vi "DoE_Control_Main.vi"() -> ()   [LabVIEW 2015]
uses:
  --Controls and TypeDefs--/DoE_Control_Cluster.ctl
  <instrlib>/JULABO DeviceDriver/Examples/Julabo Serial Control.ctl
  <instrlib>/JULABO DeviceDriver/JULABO DeviceDriver.lvlib
  <vilib>/ptbypt/NI_PtbyPt.lvlib
panel:
  out "Producer Iteration":i32
  out "Error?":bool
  out "Error?":errorcluster
  out "error out":errorcluster
  out "Measurement Iteration":i32
  out "Consumer Iteration":i32
  out "Slave Data Cluster":T1={"Current DoE"=[], "SSI 1 Flow Rate"=0.0, "SSI 2 Flow Rate"=0.0, "FLOM 1 Flow Rate"=0.0, "FLOM 2 Flow Rate"=0.0, "Pumps Running?"=FALSE, "Boolean 2"=FALSE, "Boolean 3"=FALSE, "Boolean 4"=FALSE, "At Equilibrium?"=FALSE, "Script Running?"=FALSE, "Current Script Iteration"=0.0, "Total Script Iterations"=0.0, "FLOM Pumps VISA"="COM2", "SSI 1 Pump VISA"="COM76", "SSI 2 Pump VISA"="COM74", "Huber Unistat VISA"="COM1", "SSI 3 Pump VISA"="COM76", "SSI 4 Pump VISA"="COM76", "SSI 4 Flow Rate"=0.0, "SSI 3 Flow Rate"=0.0, "Flow Meter 1 Rate "=0.0, "Flow Meter 2 Rate"=0.0, "Flow Meter 3 Rate"=0.0, "Flow Meter 4 Rate"=0.0, "SSI 1 Flow Setpoint"=0.0, "SSI 2 Flow Setpoint"=0.0, "SSI 3 Flow Setpoint"=0.0, "SSI 4 Flow Setpoint"=0.0, "Temperature Setpoint"=0.0, "Flow meter 3 COM"=17, "Flow meter 5 COM"=18, "Flow meter 4 COM"=19, "Flow meter 2 COM"=16, "Flow meter 1 COM"=15, "Unit"=enum."PSI", "Pressure COM"="COM6", "Julabo Setpoint"=0.0, "Julabo Control"=enum."Internal", "Overtemp"=50.0, "Subtemp"=-20.0, "HeatMax"=50, "CoolMax"=-100, "InternMax"=50.0, "InternMin"=0.0, "Upper Bandlimit"=100.0, "Lower Bandlimit"=0.0, "Julabo CF41 VISA"="COM3", "Xp (0.6K) Int"=0.6, "Tn (3s) Int"=3, "Tv (0s) Int"=0, "Dynamic (0: aperiodic) Int"=enum."aperiodic", "Xp (0.6K) Ext"=0.6, "Tn (3s) Ext"=3, "Tv (0s) Ext"=0, "XpU (0.6K) Ext"=0.6, "Julabo Serial Configuration"={"Baud Rate"=4800, "Parity"=2, "Data Bits"=7, "Stop Bits"=10, "Flow Control"=2}} {"Julabo Serial Configuration"."Flow Control" items=["None", "XON/XOFF", "RTS/CTS", "XON/XOFF & RTS/CTS", "DTR/DSR", "XON/XOFF & DTR/DSR"]; "Julabo Serial Configuration"."Stop Bits" items=["1.0"=10, "1.5"=15, "2.0"=20]; "Julabo Serial Configuration"."Data Bits" items=["7"=7, "8"=8]; "Julabo Serial Configuration"."Parity" items=["None", "Odd", "Even", "Mark", "Space"]; "Julabo Serial Configuration"."Baud Rate" items=["300"=300, "600"=600, "1200"=1200, "2400"=2400, "4800"=4800, "9600"=9600, "19200"=19200]; "XpU (0.6K) Ext" min=0.1 max=99.9; "Tv (0s) Ext" max=999; "Tn (3s) Ext" min=3 max=9999; "Xp (0.6K) Ext" min=0.1 max=99.9; "Tv (0s) Int" max=999; "Tn (3s) Int" min=3 max=9999; "Xp (0.6K) Int" min=0.1 max=99.9; "Lower Bandlimit" min=0.0 max=200.0; "Upper Bandlimit" min=0.0 max=200.0; "InternMin" format="%.2f"; "InternMax" format="%.2f"; "CoolMax" min=-100 max=0; "HeatMax" max=100; "Subtemp" format="%.2f"; "Overtemp" format="%.2f"; "Julabo Setpoint" format="%.2f"; "Current DoE" format="%0.3f"}
  in  "Sensor Readouts":T3(tab)
  out "Thermocouple T-Plots":T4(graph)
  in  "Apply Moving Average?":bool=TRUE
  out "dT/dt":cluster{"dx/dt":dbl, "dx/dt":dbl, "dx/dt":dbl}(graph)
  out "Flow Rate":T5(graph)
  out "dF/dt":T5(graph)
  in  "Apply dF/dt?":bool=TRUE
  out "Temp":T6(graph)
  out "Pressure":T7(graph)
  out "Internal Temp":dbl format="%.2f"
  out "Power":i8(slide) scale=-100.0..100.0
  out "Diagram":T8(graph)
  out "External Temp":dbl format="%.2f"
  out "Safety Temp":dbl
  out "Excess Temp Protection":dbl
  in  "Write to File?":bool
  in  "?":T9(tab)
  in  "Collect Spectra":bool
  out "Raman Spectrum":cluster{i32[], i32[]}[](graph)
  in  "Reset?":bool
  in  "Cancel Script":bool
  in  "Main Data Cluster":T1={"Current DoE"=[], "SSI 1 Flow Rate"=0.0, "SSI 2 Flow Rate"=0.0, "FLOM 1 Flow Rate"=0.0, "FLOM 2 Flow Rate"=0.0, "Pumps Running?"=FALSE, "Boolean 2"=FALSE, "Boolean 3"=FALSE, "Boolean 4"=FALSE, "At Equilibrium?"=FALSE, "Script Running?"=FALSE, "Current Script Iteration"=0.0, "Total Script Iterations"=0.0, "FLOM Pumps VISA"="COM2", "SSI 1 Pump VISA"="COM76", "SSI 2 Pump VISA"="COM74", "Huber Unistat VISA"="COM1", "SSI 3 Pump VISA"="COM76", "SSI 4 Pump VISA"="COM76", "SSI 4 Flow Rate"=0.0, "SSI 3 Flow Rate"=0.0, "Flow Meter 1 Rate "=0.0, "Flow Meter 2 Rate"=0.0, "Flow Meter 3 Rate"=0.0, "Flow Meter 4 Rate"=0.0, "SSI 1 Flow Setpoint"=0.0, "SSI 2 Flow Setpoint"=0.0, "SSI 3 Flow Setpoint"=0.0, "SSI 4 Flow Setpoint"=0.0, "Temperature Setpoint"=0.0, "Flow meter 3 COM"=17, "Flow meter 5 COM"=18, "Flow meter 4 COM"=19, "Flow meter 2 COM"=16, "Flow meter 1 COM"=15, "Unit"=enum."PSI", "Pressure COM"="COM6", "Julabo Setpoint"=0.0, "Julabo Control"=enum."Internal", "Overtemp"=50.0, "Subtemp"=-20.0, "HeatMax"=50, "CoolMax"=-100, "InternMax"=50.0, "InternMin"=0.0, "Upper Bandlimit"=100.0, "Lower Bandlimit"=0.0, "Julabo CF41 VISA"="COM3", "Xp (0.6K) Int"=0.6, "Tn (3s) Int"=3, "Tv (0s) Int"=0, "Dynamic (0: aperiodic) Int"=enum."aperiodic", "Xp (0.6K) Ext"=0.6, "Tn (3s) Ext"=3, "Tv (0s) Ext"=0, "XpU (0.6K) Ext"=0.6, "Julabo Serial Configuration"={"Baud Rate"=4800, "Parity"=2, "Data Bits"=7, "Stop Bits"=10, "Flow Control"=2}} {"Julabo Serial Configuration"."Flow Control" items=["None", "XON/XOFF", "RTS/CTS", "XON/XOFF & RTS/CTS", "DTR/DSR", "XON/XOFF & DTR/DSR"]; "Julabo Serial Configuration"."Stop Bits" items=["1.0"=10, "1.5"=15, "2.0"=20]; "Julabo Serial Configuration"."Data Bits" items=["7"=7, "8"=8]; "Julabo Serial Configuration"."Parity" items=["None", "Odd", "Even", "Mark", "Space"]; "Julabo Serial Configuration"."Baud Rate" items=["300"=300, "600"=600, "1200"=1200, "2400"=2400, "4800"=4800, "9600"=9600, "19200"=19200]; "XpU (0.6K) Ext" min=0.1 max=99.9; "Tv (0s) Ext" max=999; "Tn (3s) Ext" min=3 max=9999; "Xp (0.6K) Ext" min=0.1 max=99.9; "Tv (0s) Int" max=999; "Tn (3s) Int" min=3 max=9999; "Xp (0.6K) Int" min=0.1 max=99.9; "Lower Bandlimit" min=0.0 max=200.0; "Upper Bandlimit" min=0.0 max=200.0; "InternMin" format="%.2f"; "InternMax" format="%.2f"; "CoolMax" min=-100 max=0; "HeatMax" max=100; "Subtemp" format="%.2f"; "Overtemp" format="%.2f"; "Julabo Setpoint" format="%.2f"; "Current DoE" format="%0.3f"}
  in  "?":T10(tab)
  in  "Huber Unistat VISA":refnum<visa-resource-name>="COM1"
  in  "SSI 4 Pump VISA":refnum<visa-resource-name>="COM10"
  in  "SSI 2 Pump VISA 2":refnum<visa-resource-name>="COM8"
  in  "SSI 1 Pump VISA":refnum<visa-resource-name>="COM7"
  in  "FLOM Pumps VISA":refnum<visa-resource-name>="LPT1"
  in  "SSI 3 Pump VISA":refnum<visa-resource-name>="COM9"
  in  "Set COMs":bool
  out "Data_noRaman path":path caption="selected path"
  out "Data_Reactant 1 path":path caption="selected path"
  out "Data_Product path":path caption="selected path"
  out "Data_Reactant 3 path":path caption="selected path"
  out "Data_Reactant 2 path":path caption="selected path"
  out "Raman Data Path":T11
  in  "Flow meter 5 COM":u16=18
  in  "Flow meter 4 COM":u16=19
  in  "Flow meter 3 COM":u16=17
  in  "Flow meter 2 COM":u16=16
  in  "Flow meter 1 COM":u16=15
  in  "Unit":T12(ring)
  in  "Pressure COM":refnum<visa-resource-name>="COM6"
  in  "Julabo Serial Configuration":T2={"Baud Rate"=4800, "Parity"=2, "Data Bits"=7, "Stop Bits"=10, "Flow Control"=2} {"Flow Control" items=["None", "XON/XOFF", "RTS/CTS", "XON/XOFF & RTS/CTS", "DTR/DSR", "XON/XOFF & DTR/DSR"]; "Stop Bits" items=["1.0"=10, "1.5"=15, "2.0"=20]; "Data Bits" items=["7"=7, "8"=8]; "Parity" items=["None", "Odd", "Even", "Mark", "Space"]; "Baud Rate" items=["300"=300, "600"=600, "1200"=1200, "2400"=2400, "4800"=4800, "9600"=9600, "19200"=19200]}
  in  "Julabo CF41 VISA":refnum<visa-resource-name>="COM11"
  in  "RS485-Address (128: RS232)":u32=128
  in  "Create DoE":bool
  out "file write cancelled":bool caption="cancelled"
  out "written file already exists (and overwritten)":bool caption="exists"
  in  "Input DoE Values":string[][](table)
  in  "Load DoE":bool
  out "Current DoE":dbl[][](array[numeric]) format="%0.3f"
  out "DoE Filename":path
  in  "Get Current DoE":bool
  in  "Stop-Start SSI 4":bool
  in  "Stop-Start SSI 3":bool
  in  "Edit or Run/Stop SSI 4":string(combo)="Run/Stop"
  in  "Edit or Run/Stop SSI 3":string(combo)="Run/Stop"
  in  "Pump 4 (Green)?":bool
  in  "Pump 3 (Yellow)?":bool
  in  "SSI  4 (Green)":dbl
  in  "SSI  3 (Yellow)":dbl
  in  "SSI  1 (Red)":dbl
  in  "Manual Pump Control?":bool
  in  "SSI  2 (Blue)":dbl
  in  "Pump 1 (Red)?":bool
  in  "Pump 2 (Blue)?":bool
  in  "Edit or Run/Stop SSI 2":string(combo)="Run/Stop"
  in  "Edit or Run/Stop SSI 1":string(combo)="Run/Stop"
  in  "Stop-Start SSI 1":bool
  in  "Stop-Start SSI 2":bool
  in  "FLOM 1":dbl min=0.0 max=9900.0 step=1.0
  in  "FLOM 2":dbl min=0.0 max=9900.0 step=1.0
  in  "FLOM 1?":bool
  in  "FLOM 2?":bool
  in  "Stop   Start FLOM 1":bool
  in  "Stop   Start FLOM 2":bool
  in  "Edit Values, or Run Flow? FLOM 2":string(combo)="Run/Stop"
  in  "Edit Values, or Run Flow? FLOM 1":string(combo)="Run/Stop"
  out "SSI  2  (Blue) Feedback":i32 format="%.2f"
  out "SSI  1  (Red) Feedback":i32 format="%.2f"
  out "SSI  3  (Yellow) Feedback":i32 format="%.2f"
  out "SSI  4  (Green) Feedback":i32 format="%.2f"
  in  "Manual Temp Control?":bool
  in  "Julabo Setpoint":dbl format="%.2f"
  in  "Julabo Control Type":enum16{"Internal", "External"}(ring)
  in  "JulaboStartStop":bool
  in  "btnAdjustWarningLevels":bool
  in  "btnAdjustCapacityLevels":bool
  in  "btnAdjustBandLimits":bool
  in  "btnAdjustInternalTempLimits":bool
  in  "btnAdjustInternalControlParams":bool
  in  "btnAdjustExternalControlParams":bool
  in  "Xp (0.6K)":dbl=0.6 min=0.1 max=99.9
  in  "Tn (3s)":u16=3 min=3 max=9999
  in  "Tv (0s)":u16 max=999
  in  "Dynamic (0: aperiodic)":enum16{"aperiodic", "standard"}(ring)
  in  "XpU (0.6K) Ext":dbl=0.6 min=0.1 max=99.9
  in  "Xp (0.6K) Ext":dbl=0.6 min=0.1 max=99.9
  in  "Tn (3s) Ext":u16=3 min=3 max=9999
  in  "Tv (0s) Ext":u16 max=999
  in  "Overtemp":dbl=50.0 format="%.2f"
  in  "Subtemp":dbl=-20.0 format="%.2f"
  in  "HeatMax":u8=50 max=100
  in  "CoolMax":i8=-100 min=-100 max=0
  in  "InternMax":dbl=50.0 format="%.2f"
  in  "InternMin":dbl format="%.2f"
  in  "Lower Bandlim":dbl min=0.0 max=200.0
  in  "Upper Bandlim":dbl=100.0 min=0.0 max=200.0
  in  "Run Current DoE":bool
  out "Current Experiment":dbl[](array[numeric])
  in  "Debugging / Send Command":string
  in  "Debug":bool
  out "Total Script Iterations":i32
  out "Total Script Iterations 2":dbl
  out "Current Script Iteration":dbl
  out "Program State":string
  in  "STOP":bool
  # "Most recent update: 4/13/2016 - JMW"
  # "Features To-Implement:\n\n- Yield Plotting and Analytics\n- Feedback Control based on Yield\n- Error Generation System\n     - for system and user safety"
  # "Notes:\n- when starting a DoE, either have both pumps and chiller on or off\n- Always use Stop Program rather than the LabView stop button, else the Sensirion DLL\n   calls will error out and LabView must be restarted"
  # "Julabo"
  # "Limits"
  # "PID Control Parameters"
  # "Julabo"
  # "Limits"
  # "PID Control Parameters"
  # "control type \n(hold, equil)"
  # "SSI 1"
  # "SSI 2"
  # "SSI 3"
  # "SSI 4"
  # "Temp"
  # "Time"
  # "FLOM 1"
  # "FLOM 2"
  # "hold - time\nequil - watch var, deriv.\nequil timeout\n\nadd setpoint limit control"
  # "SSI 1"
  # "SSI 2"
  # "SSI 3"
  # "SSI 4"
  # "FLOM 1"
  # "FLOM 2"
  # "Temp"
  # "Time"
  # "All flow rates in increments of 10uL/min"
  # "Note: don't repeatedly turn off and on temperature control as this can wear out the compressor too rapidly according to Unistat\nManual"
  # "Gratuitously Large Power Button"
  # "Internal parameters"
  # "External parameters"
  # "Time"
  # "Control"
  # "Temp"
  # "SSI 1"
  # "SSI 2"
  # "SSI 3"
  # "SSI 4"
  # "FLOM 1"
  # "FLOM 2"
  # "uL/min , degrees C, seconds"
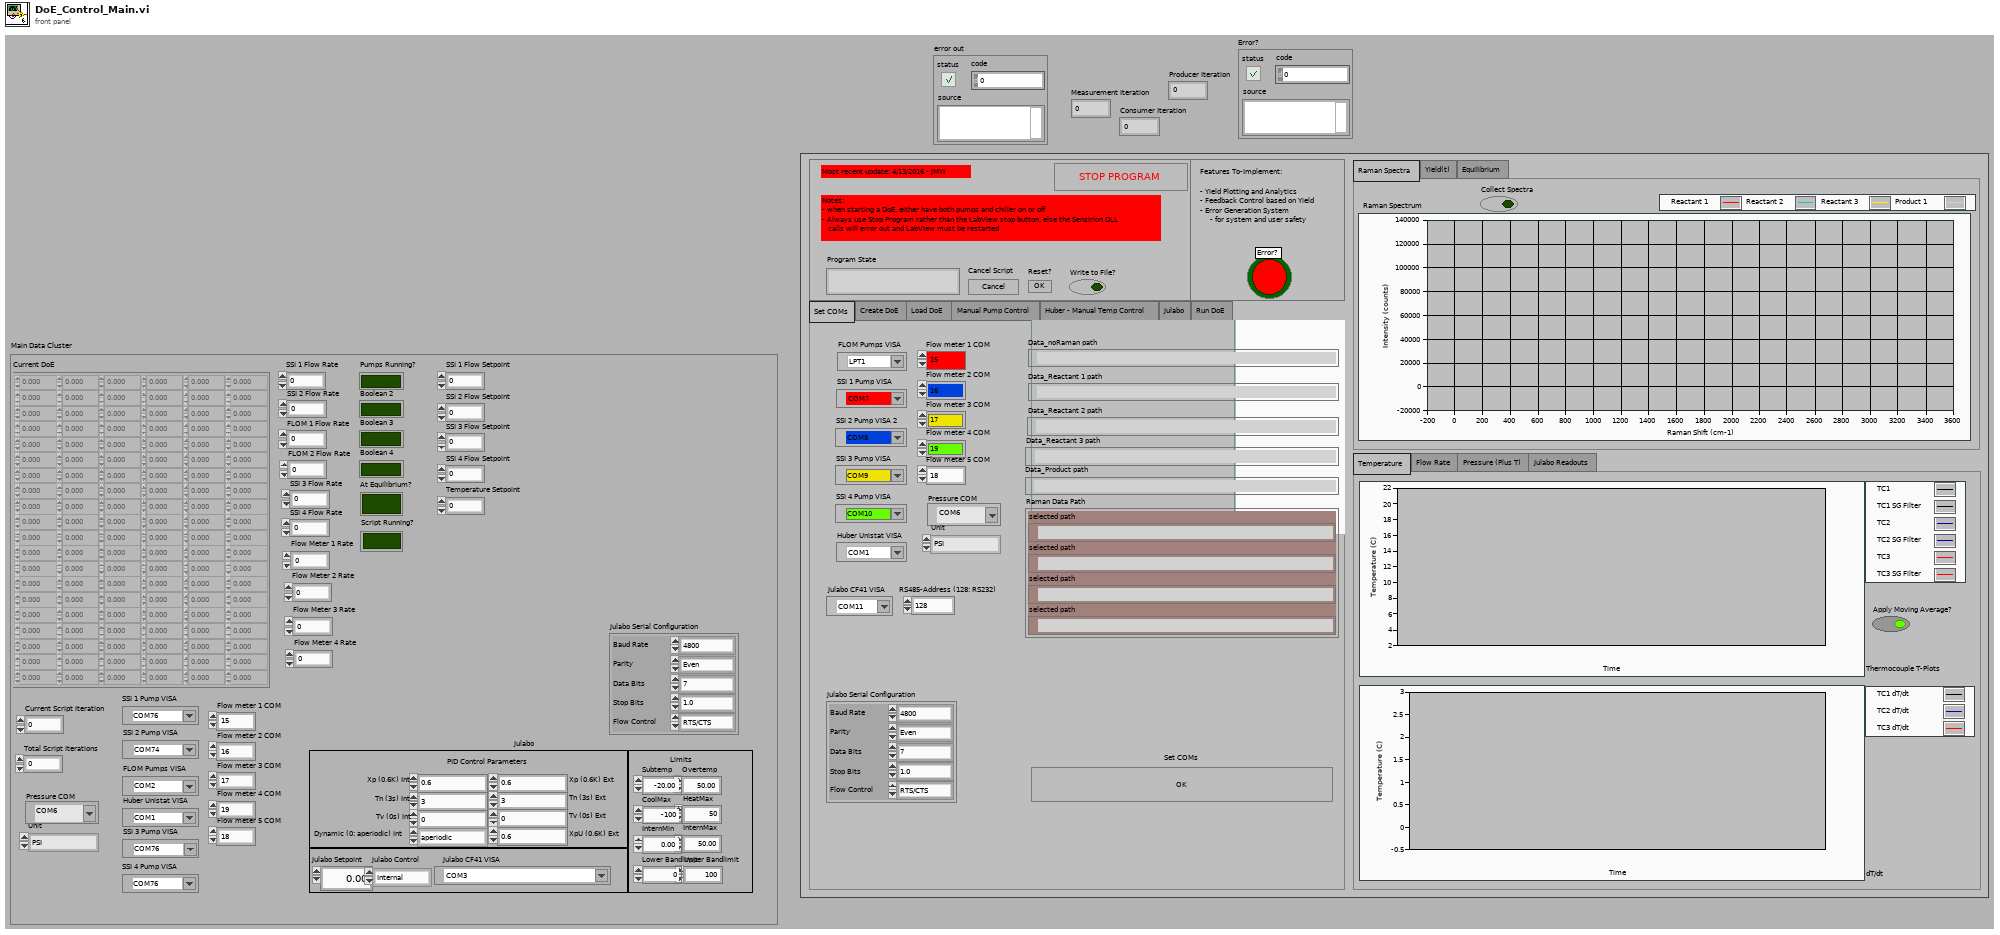
[diagram p1: front panel]
types:
  T1 = typedef "DoE_Control_Cluster.ctl" = cluster{"Current DoE":dbl[][], "SSI 1 Flow Rate":dbl, "SSI 2 Flow Rate":dbl, "FLOM 1 Flow Rate":dbl, "FLOM 2 Flow Rate":dbl, "Pumps Running?":bool, "Boolean 2":bool, "Boolean 3":bool, "Boolean 4":bool, "At Equilibrium?":bool, "Script Running?":bool, "Current Script Iteration":dbl, "Total Script Iterations":dbl, "FLOM Pumps VISA":refnum<visa-resource-name>, "SSI 1 Pump VISA":refnum<visa-resource-name>, "SSI 2 Pump VISA":refnum<visa-resource-name>, "Huber Unistat VISA":refnum<visa-resource-name>, "SSI 3 Pump VISA":refnum<visa-resource-name>, "SSI 4 Pump VISA":refnum<visa-resource-name>, "SSI 4 Flow Rate":dbl, "SSI 3 Flow Rate":dbl, "Flow Meter 1 Rate ":dbl, "Flow Meter 2 Rate":dbl, "Flow Meter 3 Rate":dbl, "Flow Meter 4 Rate":dbl, "SSI 1 Flow Setpoint":dbl, "SSI 2 Flow Setpoint":dbl, "SSI 3 Flow Setpoint":dbl, "SSI 4 Flow Setpoint":dbl, "Temperature Setpoint":dbl, "Flow meter 3 COM":u16, "Flow meter 5 COM":u16, "Flow meter 4 COM":u16, "Flow meter 2 COM":u16, "Flow meter 1 COM":u16, "Unit":enum16{"PSI", "Bar", "cm H2O", "ft H2O", "hectoPascal", "in Hg", "in H2O", "kiloPascal", "milliBar", "mmHg", "MegaPascal", "Numeric Pressure"}, "Pressure COM":refnum<visa-resource-name>, "Julabo Setpoint":dbl, "Julabo Control":enum16{"Internal", "External"}, "Overtemp":dbl, "Subtemp":dbl, "HeatMax":u8, "CoolMax":i8, "InternMax":dbl, "InternMin":dbl, "Upper Bandlimit":dbl, "Lower Bandlimit":dbl, "Julabo CF41 VISA":refnum<visa-resource-name>, "Xp (0.6K) Int":dbl, "Tn (3s) Int":u16, "Tv (0s) Int":u16, "Dynamic (0: aperiodic) Int":enum16{"aperiodic", "standard"}, "Xp (0.6K) Ext":dbl, "Tn (3s) Ext":u16, "Tv (0s) Ext":u16, "XpU (0.6K) Ext":dbl, "Julabo Serial Configuration":T2}
  T2 = typedef "Julabo Serial Control.ctl" = cluster{"Baud Rate":u32, "Parity":u16, "Data Bits":u16, "Stop Bits":u16, "Flow Control":u16}
  T3 = enum32{"Temperature", "Flow Rate", "Pressure (Plus T)", "Julabo Readouts"}
  T4 = cluster{dbl, "Filtered x":dbl, dbl, "Filtered x":dbl, dbl, "Filtered x":dbl}
  T5 = cluster{"MeasureResult Scaled":dbl, "MeasureResult Scaled":dbl, "MeasureResult Scaled":dbl, "MeasureResult Scaled":dbl, "MeasureResult Scaled":dbl}
  T6 = cluster{"Current Temperature":dbl, "Current Temperature":dbl, "Current Temperature":dbl, "Current Temperature":dbl}
  T7 = cluster{"Current Pressure":dbl, "Current Pressure":dbl, "Current Pressure":dbl, "Current Pressure":dbl}
  T8 = cluster{"Setpoint (out)":dbl, "InternalTemp (out)":dbl, "ExternalTemp (out)":dbl, "Capacity (out)":i8}
  T9 = enum32{"Raman Spectra", "Yield(t)", "Equilibrium"}
  T10 = enum32{"Set COMs", "Create DoE", "Load DoE", "Manual Pump Control", "Huber - Manual Temp Control", "Julabo", "Run DoE"}
  T11 = cluster{"selected path":path, "selected path":path, "selected path":path, "selected path":path}
  T12 = enum16{"PSI", "Bar", "cm H2O", "ft H2O", "hectoPascal", "in Hg", "in H2O", "kiloPascal", "milliBar", "mmHg", "MegaPascal", "Numeric Pressure"}
  T13 = cluster{"Array":dbl[], "Array 2":dbl[], "Array 3":dbl[], "Array 4":dbl[], "Array 5":dbl[]}
  T14 = cluster{"appended path":path, "appended path":path, "appended path":path, "appended path":path, "appended path":path}
  T15 = cluster{dbl, "Filtered x":dbl, dbl, "Filtered x":dbl, dbl, "Filtered x":dbl}[]
  T16 = cluster{"MeasureResult Scaled":dbl, "MeasureResult Scaled":dbl, "MeasureResult Scaled":dbl, "MeasureResult Scaled":dbl, "MeasureResult Scaled":dbl}[]
  T17 = cluster{"Current Pressure":dbl, "Current Pressure":dbl, "Current Pressure":dbl, "Current Pressure":dbl}[]
  T18 = cluster{"Current Temperature":dbl, "Current Temperature":dbl, "Current Temperature":dbl, "Current Temperature":dbl}[]
  T19 = cluster{"status":bool, "code":i32, "Error Report":string}
  T20 = cluster{"dx/dt":dbl, "dx/dt":dbl, "dx/dt":dbl, "dx/dt":dbl, "dx/dt":dbl}
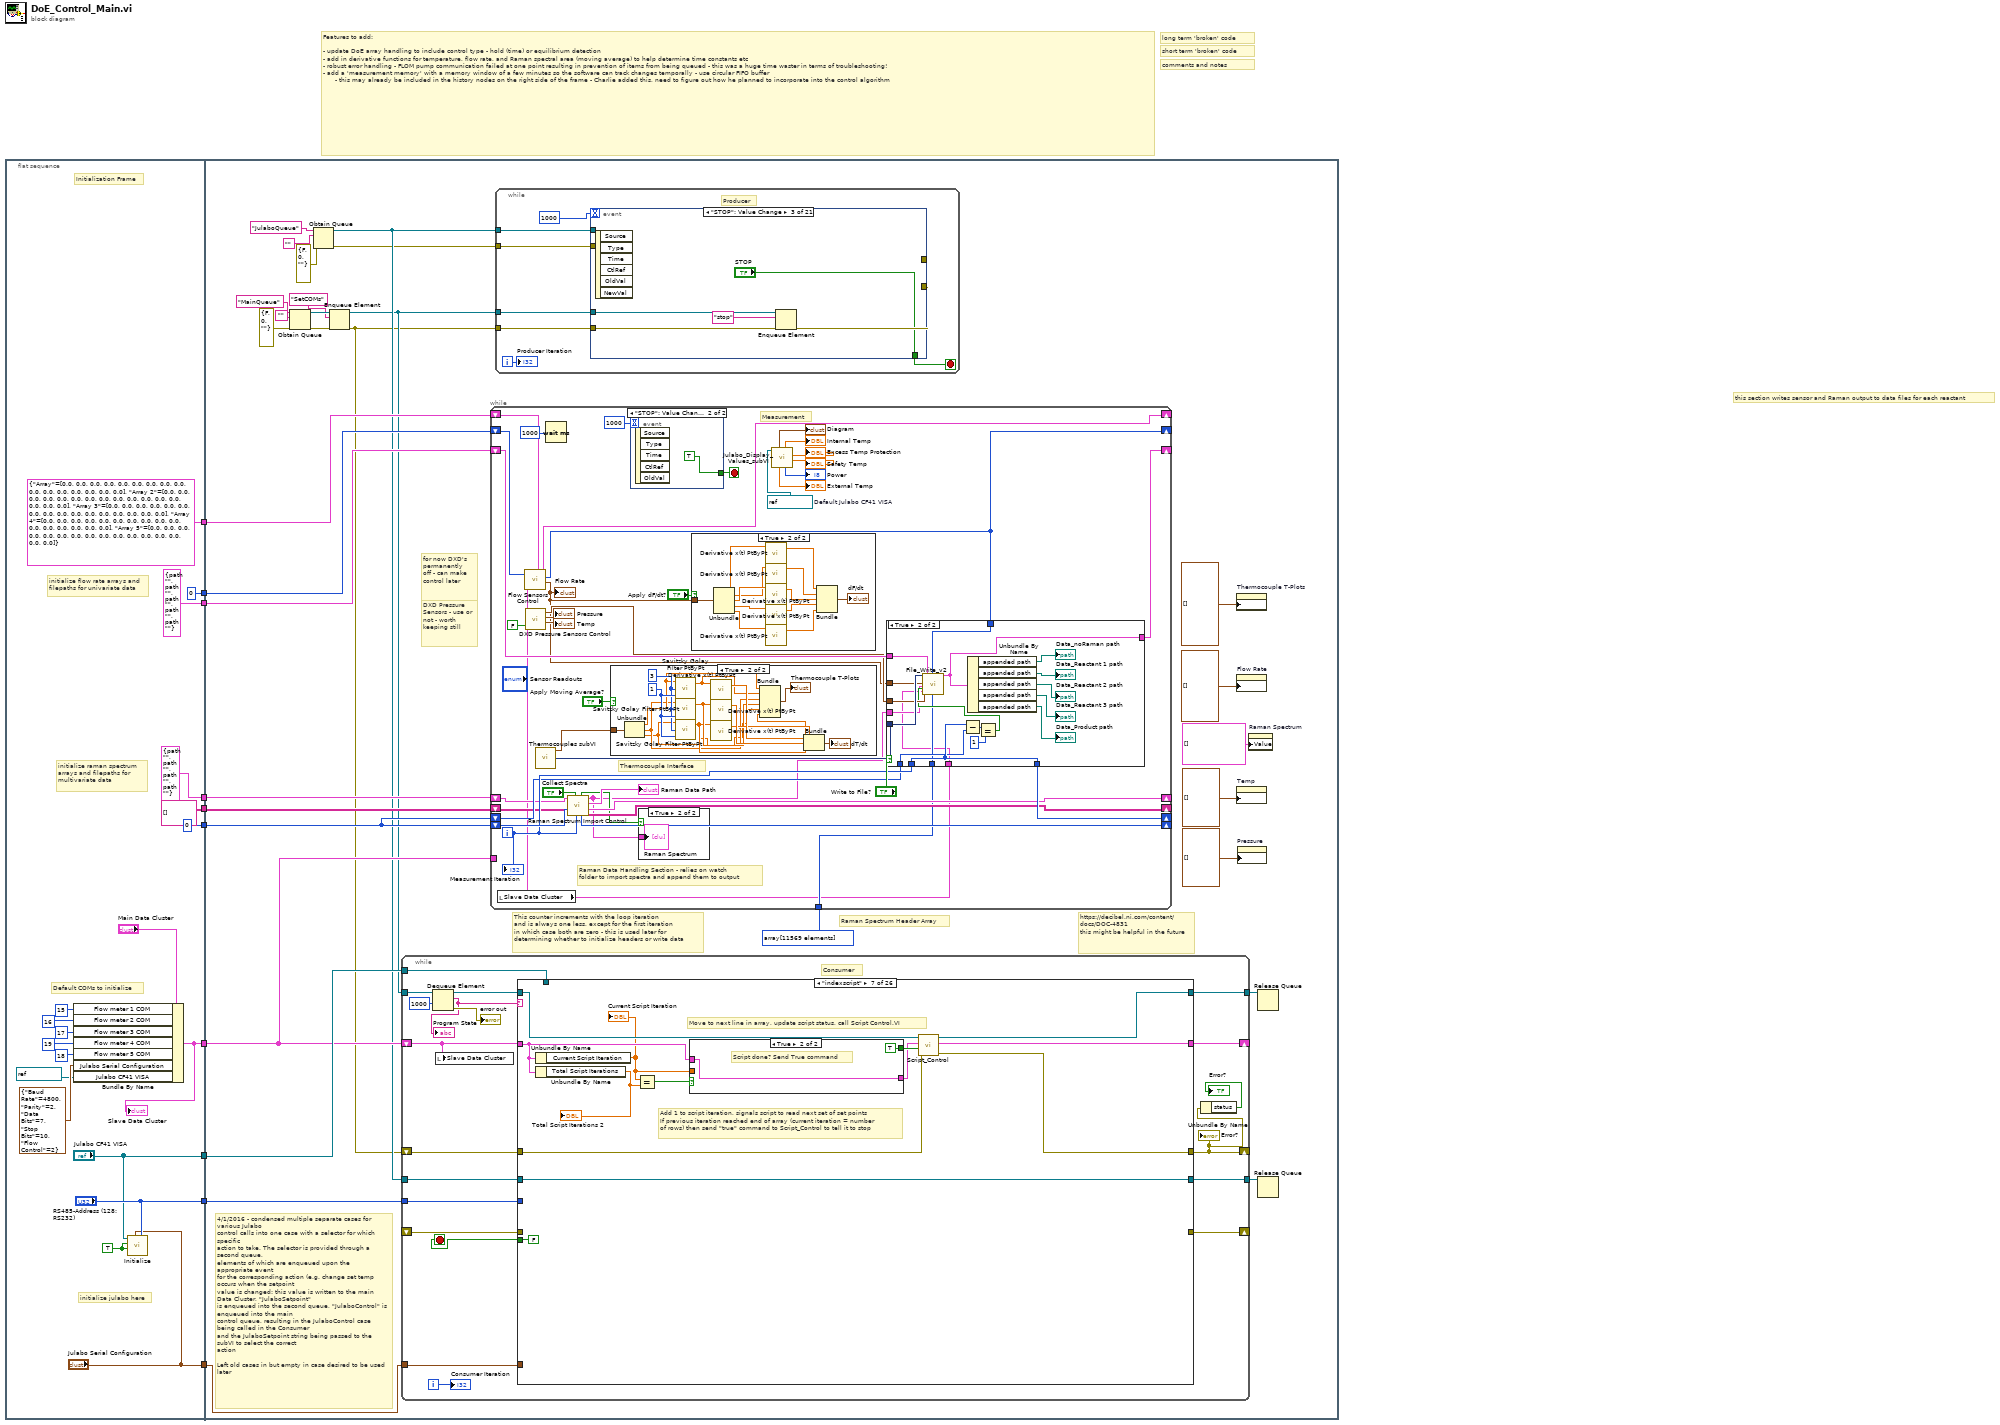
[diagram p0: block diagram]
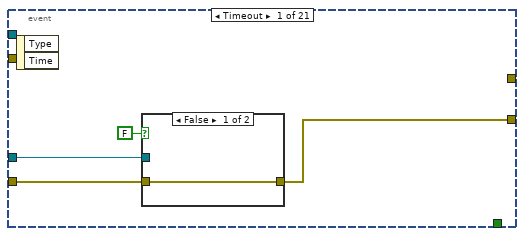
[diagram p2: hidden frame]
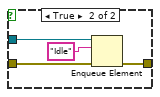
[diagram p3: hidden frame]
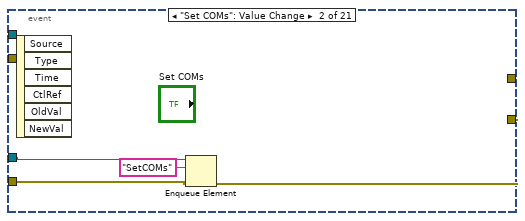
[diagram p4: hidden frame]
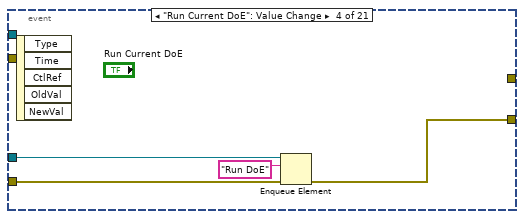
[diagram p5: hidden frame]
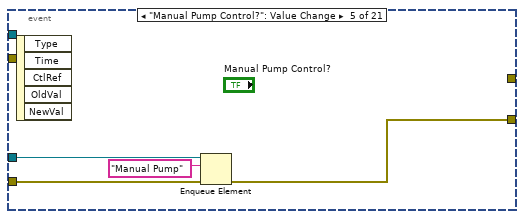
[diagram p6: hidden frame]
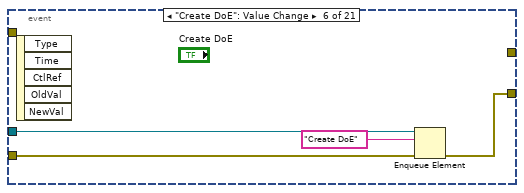
[diagram p7: hidden frame]
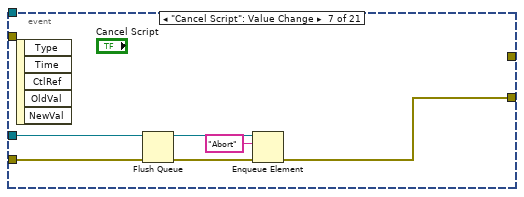
[diagram p8: hidden frame]
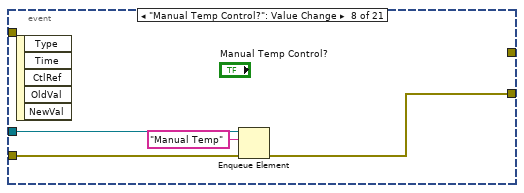
[diagram p9: hidden frame]
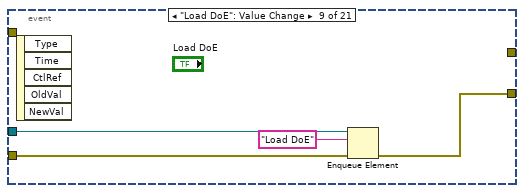
[diagram p10: hidden frame]
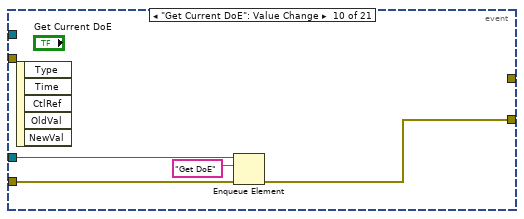
[diagram p11: hidden frame]
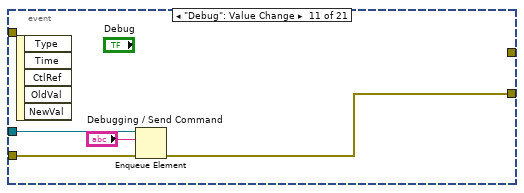
[diagram p12: hidden frame]
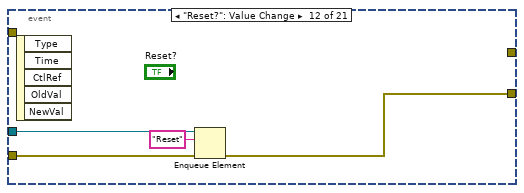
[diagram p13: hidden frame]
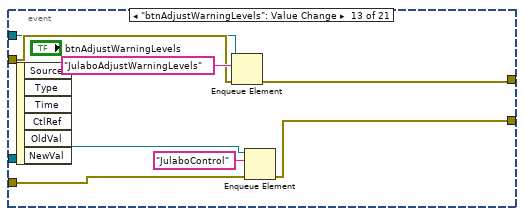
[diagram p14: hidden frame]
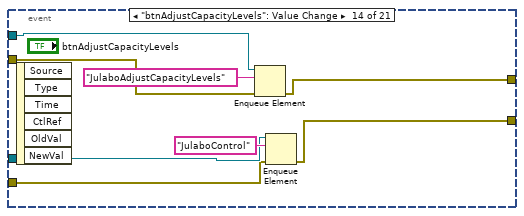
[diagram p15: hidden frame]
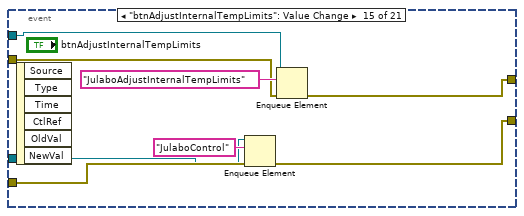
[diagram p16: hidden frame]
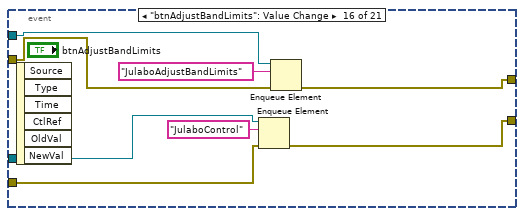
[diagram p17: hidden frame]
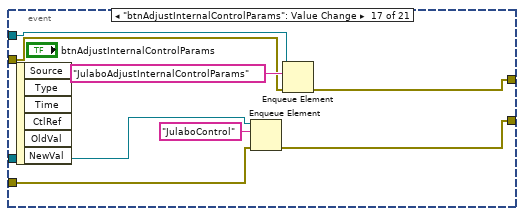
[diagram p18: hidden frame]
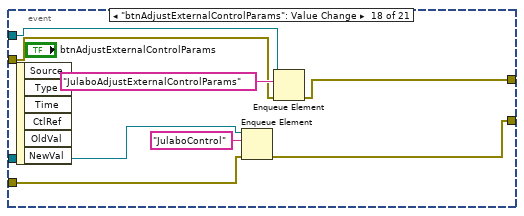
[diagram p19: hidden frame]
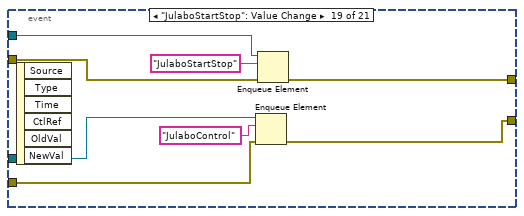
[diagram p20: hidden frame]
diagram:
  # "comments and notes"
  # "short term 'broken' code"
  # "long term 'broken' code"
  # "Features to add:\n\n- update DoE array handling to include control type - hold (time) or equilibrium detection\n- add in derivative functions for temperature, flow rate, and Raman spectral area (moving average) to help determine time constants etc\n- robust error handling - FLOM pump communication failed at one point resulting in prevention of items from being queued - this was a huge time waster in terms of troubleshooting!\n- add a 'measurement memory' with a memory window of a few minutes so the software can track changes temporally - use circular FIFO buffer\n      - this may already be included in the history nodes on the right side of the frame - Charlie added this, need to figure out how he planned to incorporate into the control algorithm"
  # "this section writes sensor and Raman output to data files for each reactant"
  n1 = flat-sequence {
    tunnel: [T11 {"selected path"=path "", "selected path"=path "", "selected path"=path "", "selected path"=path ""}] -> w10
    tunnel: [string[][] []] -> w9
    tunnel: [0] -> w8
    tunnel: ["Julabo Serial Configuration"] -> w7
    tunnel: ["RS485-Address (128: RS232)"] -> w6
    tunnel: [w18] -> w5
    tunnel: [T14 {"appended path"=path "", "appended path"=path "", "appended path"=path "", "appended path"=path "", "appended path"=path ""}] -> w4
    tunnel: [0] -> w3
    tunnel: [T13 {"Array"=[0.0, 0.0, 0.0, 0.0, 0.0, 0.0, 0.0, 0.0, 0.0, 0.0, 0.0, 0.0, 0.0, 0.0, 0.0, 0.0], "Array 2"=[0.0, 0.0, 0.0, 0.0, 0.0, 0.0, 0.0, 0.0, 0.0, 0.0, 0.0, 0.0, 0.0, 0.0, 0.0, 0.0], "Array 3"=[0.0, 0.0, 0.0, 0.0, 0.0, 0.0, 0.0, 0.0, 0.0, 0.0, 0.0, 0.0, 0.0, 0.0, 0.0, 0.0], "Array 4"=[0.0, 0.0, 0.0, 0.0, 0.0, 0.0, 0.0, 0.0, 0.0, 0.0, 0.0, 0.0, 0.0, 0.0, 0.0, 0.0], "Array 5"=[0.0, 0.0, 0.0, 0.0, 0.0, 0.0, 0.0, 0.0, 0.0, 0.0, 0.0, 0.0, 0.0, 0.0, 0.0, 0.0]}] -> w2
    tunnel: ["Julabo CF41 VISA"] -> w1
    tunnel: w10 -> [w53]
    tunnel: w9 -> [w52]
    tunnel: w8 -> [w51]
    tunnel: w7 -> [w50]
    tunnel: w6 -> [w45]
    tunnel: w5 -> [w38]
    tunnel: w4 -> [w49]
    tunnel: w3 -> [w48]
    tunnel: w2 -> [w47]
    tunnel: w1 -> [w46]
    frame #0 {
      w14 = TRUE ("ID Query? (T: Yes)")
      # "Initialization Frame"
      # "initialize julabo here"
      # "initialize raman spectrum\narrays and filepaths for\nmultivariate data"
      # "initialize flow rate arrays and\nfilepaths for univariate data"
      # "Default COMs to initialize"
      n2 = Bundle By Name(cluster="Main Data Cluster", "Flow meter 1 COM"=u16 15, "Flow meter 2 COM"=u16 16, "Flow meter 3 COM"=u16 17, "Flow meter 4 COM"=u16 19, "Flow meter 5 COM"=u16 18, "Julabo Serial Configuration"=T2 {"Baud Rate"=4800, "Parity"=2, "Data Bits"=7, "Stop Bits"=10, "Flow Control"=2}, "Julabo CF41 VISA"=refnum<visa-resource-name> "COM11") -> (w18:T1)
      "Slave Data Cluster" <- w18
      n3 = call <instrlib>:"Initialize.vi"("RS485-Address (128: RS232)"="RS485-Address (128: RS232)", "Serial Configuration"="Julabo Serial Configuration", "Reset / Default (T: Both)"=w14, "ID Query? (T: Yes)"=w14, "VISA resource name"="Julabo CF41 VISA") -> ()  [unwired: 5 in, 2 out]
    }
    frame #1 {
      # "DXD Pressure Sensors - use or not - worth keeping still"
      # "for now DXD's \npermanently\noff - can make\ncontrol later"
      # "4/1/2016 - condensed multiple separate cases for various Julabo\ncontrol calls into one case with a selector for which specific \naction to take. The selector is provided through a second queue,\nelements of which are enqueued upon the appropriate event\nfor the corresponding action (e.g. change set temp occurs when the setpoint\nvalue is changed: this value is written to the main Data Cluster, \"JulaboSetpoint\" \nis enqueued into the second queue, \"JulaboControl\" is enqueued into the main\ncontrol queue, resulting in the JulaboControl case being called in the Consumer\nand the JulaboSetpoint string being passed to the subVI to select the correct\naction\n\nLeft old cases in but empty in case desired to be used later"
      # "This counter increments with the loop iteration\nand is always one less, except for the first iteration\nin which case both are zero - this is used later for \ndetermining whether to initialize headers or write data"
      # "Raman Spectrum Header Array"
      # "https://decibel.ni.com/content/docs/DOC-4831\nthis might be helpful in the future"
      n4 = Obtain Queue(name (unnamed)="MainQueue", element data type="", error in (no error)=errorcluster {"status"=FALSE, "code"=0, "source"=""}) -> (queue out=w37:refnum<queue>, error out=w35:errorcluster)  [unwired: 2 in, 1 out]
      n5 = Obtain Queue(name (unnamed)="JulaboQueue", element data type="", error in (no error)=errorcluster {"status"=FALSE, "code"=0, "source"=""}) -> (queue out=w34:refnum<queue>, error out=w33:errorcluster)  [unwired: 2 in, 1 out]
      n6 = Enqueue Element(queue=w37, element="SetCOMs", error in (no error)=w35) -> (queue out=w32:refnum<queue>, error out=w31:errorcluster)  [unwired: 1 in, 1 out]
      n7 = while {
        shift-right: [w287] -> _
        shift-left: w31 -> [w304]
        shift-right: [w301] -> _
        shift-left: w38 -> [w300]
        tunnel: w32 -> [w305]
        tunnel: [w302] -> w60
        shift-right: [w299] -> _
        shift-left: _ -> [w298]
        tunnel: w34 -> [w289]
        tunnel: [w297] -> w54
        tunnel: w50 -> [w290]
        tunnel: w46 -> [w296]
        tunnel: w45 -> [w295]
        i -> [w294]
        stop <- w293 stop-if-true
        # "Consumer"
        n8 = Dequeue Element(queue=w305, timeout in ms (-1)=1000) -> (queue out=w303:refnum<queue>, element=w288:string, error out=→"error out":errorcluster)  [unwired: 1 in, 1 out]
        "Program State" <- w288
        n9 = local write "Slave Data Cluster"(w300) -> ()
        n10 = case shown="\"indexscript\"" w288 {
          selector: w288 -> [_ _ _ _ _ _ _ _ _ _ _ _ _ _ _ _ _ _ _ _ _ _ _ w633 _ _]
          tunnel: w304 -> [w308 w320 w325 w374 w381 w394 w405 w417 w428 w443 w462 w503 w530 w534 w537 _ _ _ _ _ _ _ _ _ _ _]
          tunnel: [w308 w320 w325 w356 w380 w393 w404 w417 w428 w433 w461 w489 w529 w534 w537 _ _ _ _ _ _ _ _ _ _ _] -> w287
          tunnel: w300 -> [w310 w321 w326 w338 w385 w389 w403 w418 w426 w431 w448 w488 w521 w536 w544 w563 w572 _ _ _ _ _ _ w631 _ _]
          tunnel: [w310 w315 w326 w333 w382 w388 w398 w418 w424 w431 w447 w488 w523 w536 w544 w565 w571 _ _ _ _ _ _ w632 _ _] -> w301
          tunnel: [w309 w319 w327 w357 w377 w392 w406 w419 w427 w432 w463 w490 w531 w535 w545 w564 w576 w611 w614 w617 w620 w623 w626 w634 w637 w640] -> w302
          tunnel: w303 -> [w309 w319 w327 w357 w379 w391 w407 w419 w427 w444 w463 w490 w531 w535 w545 w564 w576 w611 w614 w617 w620 w623 w626 w634 w637 w640]
          tunnel: [FALSE FALSE FALSE FALSE FALSE FALSE FALSE TRUE FALSE FALSE FALSE FALSE FALSE FALSE FALSE FALSE FALSE FALSE FALSE FALSE FALSE FALSE FALSE FALSE FALSE FALSE] -> w293
          tunnel: [_ _ _ _ _ _ _ _ _ _ _ _ _ _ _ _ w574 _ _ _ _ _ _ _ _ _] -> w299
          tunnel: w298 -> [_ _ _ _ _ _ _ _ _ _ _ _ _ _ _ _ _ _ _ _ _ _ _ _ _ _]
          tunnel: w289 -> [w306 w311 w323 w331 w375 w386 w395 w415 w420 w429 w449 w474 w512 w532 w538 w546 w567 w609 w612 w615 w618 w621 w624 w627 w635 w638]
          tunnel: [w306 w311 w323 w331 w375 w386 w395 w415 w420 w429 w449 w474 w512 w532 w538 w546 w566 w609 w612 w615 w618 w621 w624 w627 w635 w638] -> w297
          tunnel: w290 -> [_ _ _ _ _ _ _ _ _ _ _ _ _ _ _ w549 _ _ _ _ _ _ _ _ _ _]
          tunnel: w296 -> [_ _ _ _ _ _ _ _ _ _ _ _ _ _ _ w548 _ _ _ _ _ _ _ _ _ _]
          tunnel: w295 -> [_ _ _ _ _ _ _ _ _ _ _ _ _ _ _ _ _ _ _ _ _ _ _ _ _ _]
          frame "Initialize" {
            # "Generic Error"
            # "Julabo Error"
          }
          frame "Load DoE" {
            n11 = call "DoE_Read_Standalone.vi"() -> ("all rows"=w318:dbl[][], "new file path (Not A Path if cancelled)"=→"DoE Filename":path)  [unwired: 14 in]
            "Current DoE" <- w318
            n12 = Array Size(array=w318) -> (size(s)=w316:i32[])
            n13 = Index Array(array=w316, index #2=0 ("index")) -> (element #2=w314:i32)  [unwired: 1 in, 1 out]
            "Total Script Iterations" <- w314
            n14 = Bundle By Name(cluster=w321, "Current DoE"=w318) -> (w317:T1)
            n15 = Bundle By Name(cluster=w317, "Total Script Iterations"=w314) -> (w315:T1)
          }
          frame "Create DoE" {
            n16 = call "DoE_Create_Standalone.vi"("Input DoE Values"="Input DoE Values") -> ("written file already exists (and overwritten)"=→"written file already exists (and overwritten)":bool, "file write cancelled"=→"file write cancelled":bool)  [unwired: 9 in]
          }
          frame "Manual Pump" {
            n17 = Unbundle By Name(w338) -> ("FLOM Pumps VISA"=w355:refnum<visa-resource-name>, "SSI 1 Pump VISA"=w354:refnum<visa-resource-name>, "SSI 2 Pump VISA"=w353:refnum<visa-resource-name>, "SSI 3 Pump VISA"=w350:refnum<visa-resource-name>, "SSI 4 Pump VISA"=w349:refnum<visa-resource-name>)  [unwired: 1 out]
            n18 = call "Series I Pump Flow Write SubVI both pumps standalone.vi"("Write to Pump 1?"="Pump 1 (Red)?", "Write to Pump 2?"="Pump 2 (Blue)?", "Edit or Run/Stop Series IA Pump"="Edit or Run/Stop SSI 1", "Stop-Start"="Stop-Start SSI 1", "Pump IA Flow Rate (10uL/min)"="SSI  1 (Red)", "Stop-Start 2"="Stop-Start SSI 2", "error in (no error)"=w374, "Pump 1B Flow Rate (10uL/min)"="SSI  2 (Blue)", "Edit or Run/Stop Series IB Pump"="Edit or Run/Stop SSI 2", "Series IA Pump VISA"=w354, "Series IB Pump VISA"=w353) -> ("Pump 1A flow rate Out"=→"SSI  1  (Red) Feedback":i32, "Pump 1B flow rate Out"=→"SSI  2  (Blue) Feedback":i32, "Error Out"=w352:T19)  [unwired: 13 in, 1 out]
            n19 = call "Series I Pump Flow Write SubVI both pumps standalone.vi"("Write to Pump 1?"="Pump 3 (Yellow)?", "Write to Pump 2?"="Pump 4 (Green)?", "Edit or Run/Stop Series IA Pump"="Edit or Run/Stop SSI 3", "Stop-Start"="Stop-Start SSI 3", "Pump IA Flow Rate (10uL/min)"="SSI  3 (Yellow)", "Stop-Start 2"="Stop-Start SSI 4", "error in (no error)"=w352, "Pump 1B Flow Rate (10uL/min)"="SSI  4 (Green)", "Edit or Run/Stop Series IB Pump"="Edit or Run/Stop SSI 4", "Series IA Pump VISA"=w350, "Series IB Pump VISA"=w349) -> ("Pump 1A flow rate Out"=→"SSI  3  (Yellow) Feedback":i32, "Pump 1B flow rate Out"=→"SSI  4  (Green) Feedback":i32, "Error Out"=w351:T19)  [unwired: 13 in, 1 out]
            n20 = Bundle By Name(cluster=w338, "SSI 1 Flow Setpoint"="SSI  1 (Red)", "SSI 2 Flow Setpoint"="SSI  2 (Blue)", "SSI 3 Flow Setpoint"="SSI  3 (Yellow)", "SSI 4 Flow Setpoint"="SSI  4 (Green)") -> (w333:T1)
            n21 = call "FLOM Pump Flow Write SubVI - standalone.vi"("Write to Pump 1?"="FLOM 1?", "Write to Pump 2?"="FLOM 2?", "Mode"="Continuous Flow", "Edit Values, or Run Flow?\n(Only for Continuous Flow)"="Edit Values, or Run Flow? FLOM 1", "Stop   Start"="Stop   Start FLOM 1", "Pump 1 Flow Rate (uL/min)"="FLOM 1", "Stop   Start 2"="Stop   Start FLOM 2", "error in (no error) 2"=w351, "Pump 2 Flow Rate (uL/min)"="FLOM 2", "Mode 2"="Continuous Flow", "Edit Values, or Run Flow?\n(Only for Continuous Flow) 2"="Edit Values, or Run Flow? FLOM 2", "VISA resource"=w355) -> ("Error Out"=w356:T19)  [unwired: 14 in, 1 out]
          }
          frame "Run DoE" {
            # "start at -1 to increment to 0 for first set point"
            n22 = Bundle By Name(cluster=w385, "Script Running?"=TRUE, "Current Script Iteration"=-1.0) -> (w382:T1)
            n23 = Enqueue Element(queue=w379, element="indexscript", error in (no error)=w381) -> (queue out=w377:refnum<queue>, error out=w380:errorcluster)  [unwired: 1 in, 1 out]
          }
          frame "CheckEquilibrium" {
            # "Set to assume at\nequilibrium,\nchange later when\nalgorithm developed"
            n24 = call "CheckEquilibrium.vi"("error in (no error)"=w394, "Eventually replace this with output from an algorithm to check equilibrium"=TRUE, "queue in"=w391, "Main Data Cluster In"=w389) -> ("error out"=w393:errorcluster, "queue out"=w392:refnum<queue>, "Main Data Cluster Out"=w388:T1)  [unwired: 5 in]
          }
          frame "indexscript" {
            # "Add 1 to script iteration, signals script to read next set of set points\nIf previous iteration reached end of array (current iteration = number\nof rows) then send \"true\" command to Script_Control to tell it to stop"
            # "Move to next line in array, update script status, call Script Control.VI"
            n25 = Unbundle By Name(w403) -> ("Current Script Iteration"=w400:dbl)
            "Current Script Iteration" <- w400
            n26 = Unbundle By Name(w403) -> ("Total Script Iterations"=w401:dbl)
            "Total Script Iterations 2" <- w401
            n27 = Equal?(x=w400, y=w401) -> (x = y?=w397:bool)
            n28 = case shown="True" w397 {
              tunnel: w400 -> [w412 _]
              tunnel: w403 -> [w410 w414]
              tunnel: [w409 w414] -> w399
              tunnel: [FALSE TRUE] -> w402
              frame False {
                n29 = Increment(x=w412) -> (x+1=w411:dbl)
                n30 = Bundle By Name(cluster=w410, "Current Script Iteration"=w411) -> (w409:T1)
              }
              frame True {
                # "Script done? Send True command"
              }
            }
            n31 = call "Script_Control.vi"("error in (no error)"=w405, "Script done? Replace later"=w402, "Main Data Cluster In"=w399, "MainQueueIn"=w407) -> ("error out"=w404:errorcluster, "Main Data Cluster Out"=w398:T1, "MainQueueOut"=w406:refnum<queue>)  [unwired: 5 in]
          }
          frame "stop" {
          }
          frame "Reset" {
            n32 = Bundle By Name(cluster=w426, "At Equilibrium?"=FALSE, "Script Running?"=FALSE, "Current Script Iteration"=-1.0) -> (w424:T1)
          }
          frame "Abort" {
            n33 = Flush Queue(queue=w444, error in (no error)=w443) -> (queue out=w442:refnum<queue>, error out=w441:errorcluster)  [unwired: 1 out]
            n34 = Enqueue Element(queue=w442, element="StopPumps", error in (no error)=w441) -> (queue out=w439:refnum<queue>, error out=w440:errorcluster)  [unwired: 1 in, 1 out]
            n35 = Enqueue Element(queue=w439, element="StopTemp", error in (no error)=w440) -> (queue out=w435:refnum<queue>, error out=w436:errorcluster)  [unwired: 1 in, 1 out]
            n36 = Enqueue Element(queue=w435, element="Reset", error in (no error)=w436) -> (queue out=w432:refnum<queue>, error out=w433:errorcluster)  [unwired: 1 in, 1 out]
          }
          frame "StopPumps" {
            w454 = "Run/Stop" ("Edit or Run/Stop Series IB Pump")
            w453 = FALSE ("Stop-Start")
            w455 = TRUE ("Write to Pump 1?")
            # "for now, no FLOMs, set so as\nto not attempt to communicate"
            n37 = Unbundle By Name(w448) -> ("FLOM Pumps VISA"=w460:refnum<visa-resource-name>, "SSI 1 Pump VISA"=w459:refnum<visa-resource-name>, "SSI 2 Pump VISA"=w458:refnum<visa-resource-name>, "SSI 3 Pump VISA"=w452:refnum<visa-resource-name>, "SSI 4 Pump VISA"=w451:refnum<visa-resource-name>)
            n38 = call "Series I Pump Flow Write SubVI both pumps standalone.vi"("Write to Pump 1?"=w455, "Write to Pump 2?"=w455, "Edit or Run/Stop Series IA Pump"=w454, "Stop-Start"=w453, "Stop-Start 2"=w453, "error in (no error)"=w462, "Edit or Run/Stop Series IB Pump"=w454, "Series IA Pump VISA"=w459, "Series IB Pump VISA"=w458) -> ("Error Out"=w457:T19)  [unwired: 15 in, 3 out]
            n39 = call "Series I Pump Flow Write SubVI both pumps standalone.vi"("Write to Pump 1?"=w455, "Write to Pump 2?"=w455, "Edit or Run/Stop Series IA Pump"=w454, "Stop-Start"=w453, "Stop-Start 2"=w453, "error in (no error)"=w457, "Edit or Run/Stop Series IB Pump"=w454, "Series IA Pump VISA"=w452, "Series IB Pump VISA"=w451) -> ("Error Out"=w456:T19)  [unwired: 15 in, 3 out]
            n40 = case shown="True" FALSE {
              tunnel: [w469 w470] -> w461
              tunnel: w460 -> [w468 _]
              tunnel: w456 -> [w467 w470]
              tunnel: w455 -> [w466 _]
              tunnel: w454 -> [w465 _]
              tunnel: w453 -> [w464 _]
              frame False {
                n41 = call "FLOM Pump Flow Write SubVI - standalone.vi"("Write to Pump 1?"=w466, "Write to Pump 2?"=w466, "Edit Values, or Run Flow?\n(Only for Continuous Flow)"=w465, "Stop   Start"=w464, "Stop   Start 2"=w464, "error in (no error) 2"=w467, "Edit Values, or Run Flow?\n(Only for Continuous Flow) 2"=w465, "VISA resource"=w468) -> ("Error Out"=w469:T19)  [unwired: 18 in, 1 out]
              }
              frame True {
              }
            }
            n42 = Bundle By Name(cluster=w448, "Pumps Running?"=FALSE) -> (w447:T1)
          }
          frame "SetPumps" {
            w473 = 6  # Temp
            w472 = 7  # Time
            w480 = 5  # FLOM2
            w481 = 4  # FLOM1
            w486 = TRUE ("Write to Pump 1?")
            w487 = "Edit" ("Edit or Run/Stop Series IB Pump")
            w496 = 3  # SSI4
            w497 = 2  # SSI3
            w498 = 1  # SSI2
            w499 = 0  # SSI1
            # "no FLOMs - don't write to them"
            # "for now, no FLOMs so write-to FLOM disabled"
            # "FLOM pumps"
            # "SSI pumps"
            # "Set flow rate values to correct pumps"
            # "get one row from array"
            # "set this up to call the pump control VI's, then call the pump start command"
            # "Updates \"Current Experiment\" Indicator once pumps are set"
            n43 = Unbundle By Name(w488) -> ("Current DoE"=w502:dbl[][])
            n44 = Unbundle By Name(w488) -> ("Current Script Iteration"=w501:dbl)
            n45 = Index Array(array=w502, index (row)=w501) -> (element=w500:dbl[])  [unwired: 1 in]
            "Current Experiment" <- w500
            n46 = Unbundle By Name(w488) -> ("FLOM Pumps VISA"=w491:refnum<visa-resource-name>, "SSI 1 Pump VISA"=w493:refnum<visa-resource-name>, "SSI 2 Pump VISA"=w492:refnum<visa-resource-name>, "SSI 3 Pump VISA"=w485:refnum<visa-resource-name>, "SSI 4 Pump VISA"=w484:refnum<visa-resource-name>)  [unwired: 1 out]
            n47 = Index Array(array=w500, index #1=w499, index #2=w498, index #3=w497, index #4=w496, index #5=w481, index #6=w480, index #7=w473, index #8=w472) -> (element #1=w495:dbl, element #2=w494:dbl, element #3=w479:dbl, element #4=w478:dbl, element #5=w476:dbl, element #6=w477:dbl)  [unwired: 2 out]
            n48 = call "Series I Pump Flow Write SubVI both pumps standalone.vi"("Write to Pump 1?"=w486, "Write to Pump 2?"=w486, "Edit or Run/Stop Series IA Pump"=w487, "Pump IA Flow Rate (10uL/min)"=w495, "error in (no error)"=w503, "Pump 1B Flow Rate (10uL/min)"=w494, "Edit or Run/Stop Series IB Pump"=w487, "Series IA Pump VISA"=w493, "Series IB Pump VISA"=w492) -> ("Error Out"=w483:T19)  [unwired: 15 in, 3 out]
            n49 = call "Series I Pump Flow Write SubVI both pumps standalone.vi"("Write to Pump 1?"=w486, "Write to Pump 2?"=w486, "Edit or Run/Stop Series IA Pump"=w487, "Pump IA Flow Rate (10uL/min)"=w479, "error in (no error)"=w483, "Pump 1B Flow Rate (10uL/min)"=w478, "Edit or Run/Stop Series IB Pump"=w487, "Series IA Pump VISA"=w485, "Series IB Pump VISA"=w484) -> ("Error Out"=w482:T19)  [unwired: 15 in, 3 out]
            n50 = case shown="False" FALSE {
              tunnel: w491 -> [_ w511]
              tunnel: [w504 w510] -> w489
              tunnel: w482 -> [w504 w507]
              tunnel: w477 -> [_ w506]
              tunnel: w476 -> [_ w505]
              frame False {
              }
              frame True {
                w508 = FALSE ("Write to Pump 1?")
                w509 = "Edit" ("Edit Values, or Run Flow?\n(Only for Continuous Flow)")
                n51 = call "FLOM Pump Flow Write SubVI - standalone.vi"("Write to Pump 1?"=w508, "Write to Pump 2?"=w508, "Edit Values, or Run Flow?\n(Only for Continuous Flow)"=w509, "Pump 1 Flow Rate (uL/min)"=w505, "error in (no error) 2"=w507, "Pump 2 Flow Rate (uL/min)"=w506, "Edit Values, or Run Flow?\n(Only for Continuous Flow) 2"=w509, "VISA resource"=w511) -> ("Error Out"=w510:T19)  [unwired: 18 in, 1 out]
              }
            }
          }
          frame "StartPumps" {
            w517 = TRUE ("Stop-Start")
            w524 = TRUE ("Stop   Start")
            w525 = "Run/Stop" ("Edit Values, or Run Flow?\n(Only for Continuous Flow) 2")
            w516 = "Run/Stop" ("Edit or Run/Stop Series IB Pump")
            w518 = TRUE ("Write to Pump 1?")
            n52 = Unbundle By Name(w521) -> ("FLOM Pumps VISA"=w526:refnum<visa-resource-name>, "SSI 1 Pump VISA"=w528:refnum<visa-resource-name>, "SSI 2 Pump VISA"=w527:refnum<visa-resource-name>)
            n53 = Unbundle By Name(w521) -> ("SSI 3 Pump VISA"=w515:refnum<visa-resource-name>, "SSI 4 Pump VISA"=w514:refnum<visa-resource-name>)
            n54 = call "Series I Pump Flow Write SubVI both pumps standalone.vi"("Write to Pump 1?"=w518, "Write to Pump 2?"=w518, "Edit or Run/Stop Series IA Pump"=w516, "Stop-Start"=w517, "Stop-Start 2"=w517, "error in (no error)"=w530, "Edit or Run/Stop Series IB Pump"=w516, "Series IA Pump VISA"=w528, "Series IB Pump VISA"=w527) -> ("Error Out"=w520:T19)  [unwired: 15 in, 3 out]
            n55 = call "Series I Pump Flow Write SubVI both pumps standalone.vi"("Write to Pump 1?"=w518, "Write to Pump 2?"=w518, "Edit or Run/Stop Series IA Pump"=w516, "Stop-Start"=w517, "Stop-Start 2"=w517, "error in (no error)"=w520, "Edit or Run/Stop Series IB Pump"=w516, "Series IA Pump VISA"=w515, "Series IB Pump VISA"=w514) -> ("Error Out"=w519:T19)  [unwired: 15 in, 3 out]
            n56 = call "FLOM Pump Flow Write SubVI - standalone.vi"("Write to Pump 1?"=w518, "Write to Pump 2?"=w518, "Edit Values, or Run Flow?\n(Only for Continuous Flow)"=w525, "Stop   Start"=w524, "Stop   Start 2"=w524, "error in (no error) 2"=w519, "Edit Values, or Run Flow?\n(Only for Continuous Flow) 2"=w525, "VISA resource"=w526) -> ("Error Out"=w529:T19)  [unwired: 18 in, 1 out]
            n57 = Bundle By Name(cluster=w521, "Pumps Running?"=TRUE ("Boolean")) -> (w523:T1)
          }
          frame "Idle", Default {
          }
          frame "SetTemp" {
            (unwired) "SP@" ("Commands")
            # "Due to different control method with Julabo, this case will need to be modified!"
            # "Removed Huber subVI, replace with Julabo subVI"
            n58 = Unbundle By Name(w544) -> ("Current DoE"=w541:dbl[][])
            n59 = Unbundle By Name(w544) -> ("Current Script Iteration"=w542:dbl)
            n60 = Unbundle By Name(w544) -> ()  [unwired: 1 out]
            n61 = Index Array(array=w541, index (row)=w542) -> (element=w540:dbl[])  [unwired: 1 in]
            n62 = Index Array(array=w540, index=6) -> ()  [unwired: 1 out]
          }
          frame "SetCOMs" {
            n63 = Bundle By Name(cluster=w563, "Julabo CF41 VISA"=w548, "FLOM Pumps VISA"="FLOM Pumps VISA", "SSI 1 Pump VISA"="SSI 1 Pump VISA", "SSI 2 Pump VISA"="SSI 2 Pump VISA 2", "SSI 3 Pump VISA"="SSI 3 Pump VISA", "SSI 4 Pump VISA"="SSI 4 Pump VISA", "Huber Unistat VISA"="Huber Unistat VISA", "Pressure COM"="Pressure COM", "Unit"="Unit", "Flow meter 1 COM"="Flow meter 1 COM", "Flow meter 2 COM"="Flow meter 2 COM", "Flow meter 3 COM"="Flow meter 3 COM", "Flow meter 4 COM"="Flow meter 4 COM", "Flow meter 5 COM"="Flow meter 5 COM", "Julabo Serial Configuration"=w549) -> (w565:T1)
          }
          frame "JulaboControl" {
            n64 = flat-sequence {
              tunnel: ["JulaboStartStop"] -> w575
              tunnel: [w579] -> w573
              tunnel: w572 -> [w600]
              tunnel: [w599] -> w570
              tunnel: w567 -> [w580]
              tunnel: [w578] -> w568
              tunnel: w575 -> [w608]
              tunnel: [w607] -> w574
              tunnel: w573 -> [w606]
              tunnel: [w605] -> w571
              tunnel: w570 -> [w604]
              tunnel: [w603] -> w566
              tunnel: w568 -> [w603]
              frame #0 {
                # "Write most up-to-date values into cluster:\ncontrol subVI will pull the values needed\nfor the specific action call"
                n65 = Dequeue Element(queue=w580, timeout in ms (-1)=1000) -> (queue out=w578:refnum<queue>, element=w579:string)  [unwired: 1 in, 2 out]
                n66 = Bundle By Name(cluster=w600, "Julabo Setpoint"="Julabo Setpoint", "Julabo Control"="Julabo Control Type", "Overtemp"="Overtemp", "Subtemp"="Subtemp", "CoolMax"="CoolMax", "HeatMax"="HeatMax", "InternMin"="InternMin", "InternMax"="InternMax", "Lower Bandlimit"="Lower Bandlim", "Upper Bandlimit"="Upper Bandlim", "Xp (0.6K) Int"="Xp (0.6K)", "Tn (3s) Int"="Tn (3s)", "Tv (0s) Int"="Tv (0s)", "Dynamic (0: aperiodic) Int"="Dynamic (0: aperiodic)", "Xp (0.6K) Ext"="Xp (0.6K) Ext", "Tn (3s) Ext"="Tn (3s) Ext", "Tv (0s) Ext"="Tv (0s) Ext", "XpU (0.6K) Ext"="XpU (0.6K) Ext") -> (w599:T1)
              }
              frame #1 {
                # "not wired for now"
                n67 = Unbundle By Name(w604) -> ()  [unwired: 1 out]
                n68 = call "Doe_Julabo_Control_subVI_2.vi"("Julabo CF41 VISA"=refnum<visa-resource-name> "COM11", "Data Cluster In"=w604, "Case Selector"=w606, "StartStop"=w608) -> ("Data Cluster Out"=w605:T1, "error out 2"=w607:errorcluster)  [unwired: 10 in]
              }
            }
          }
          frame "JulaboAdjustWarningLevels" {
          }
          frame "JulaboAdjustCapacityLevels" {
          }
          frame "JulaboAdjustInternalTempLimits" {
          }
          frame "JulaboAdjustBandLimits" {
          }
          frame "JulaboAdjustInternalControlParams" {
          }
          frame "JulaboAdjustExternalControlParams" {
          }
          frame "JulaboStartStop" {
            # "This is currently not used"
            n69 = Unbundle By Name(w631) -> ("Julabo CF41 VISA"=w630:refnum<visa-resource-name>)
            n70 = call "Doe_Julabo_Control_subVI_2.vi"("Julabo CF41 VISA"=w630, "Data Cluster In"=w631, "Case Selector"=w633, "StartStop"=FALSE) -> ("Data Cluster Out"=w632:T1)  [unwired: 10 in, 1 out]
          }
          frame "JulaboControlType" {
          }
          frame "JulaboSetpoint" {
          }
        }
        "Error?" <- w287
        n71 = Unbundle By Name(w287) -> ("status"=→"Error?":bool)
        "Consumer Iteration" <- w294
      }
      n72 = while {
        shift-right: [w232] -> _
        shift-left: w51 -> [w233]
        shift-right: [w235] -> _
        shift-left: w49 -> [w223]
        shift-right: [w231] -> _
        shift-left: w51 -> [w229]
        shift-right: [w226] -> _
        shift-left: w52 -> [w225]
        shift-right: [w228] -> _
        shift-left: w53 -> [w227]
        tunnel: i32[] array[11569 elements] ("Array") -> [w224]
        shift-right: [w222] -> _
        shift-left: w47 -> [w221]
        shift-right: [w218] -> _
        shift-left: w48 -> [w220]
        tunnel: w38 -> [_]
        i -> [w230]
        stop <- w200 stop-if-true
        w203 = refnum<visa-resource-name> "COM11"  # Default Julabo CF41 VISA
        # "Measurement"
        # "Raman Data Handling Section - relies on watch \nfolder to import spectra and append them to output"
        # "Thermocouple Interface"
        n73 = local read "Slave Data Cluster"() -> (w204:T1)
        n74 = call "Flow Sensors Control.vi"("Initialized Array Cluster"=w221, "Initialized Index"=w220, "Slave Data Cluster"=w204) -> ("Flow Rate Data Out"=w196:cluster{dbl, dbl, dbl, dbl, dbl}, "Numeric out"=w218:i32, "Flow Rate Data Array Cluster Out"=w222:T13)  [unwired: 6 in]
        "Flow Rate" <- w196
        n75 = call "DXD Pressure Sensors Control.vi"("Record Pressure?"=FALSE, "Slave Data Cluster"=w204) -> ("Temperature Plot"=→"Temp":T6, "PressurePlot"=→"Pressure":T7, "Pressure Data Out to Write"=w215:T7)  [unwired: 7 in]
        n76 = call "Thermocouples subVI.vi"() -> ("data"=w219:dynamicdata, "Cluster"=w202:cluster{dbl, dbl, dbl})  [unwired: 10 in]
        n77 = Wait (ms)(milliseconds to wait=u32 1000) -> ()  [unwired: 1 out]
        n78 = call "Raman Spectrum Import Control.vi"("Iterations"=w230, "Collect Spectra"="Collect Spectra", "Numeric in"=w233, "Array in"=w225, "Cluster in"=w227) -> ("Array 3"=w226:string[][], "Cluster 3"=w228:T11, "Cluster out"=→"Raman Data Path":T11, "Array out"=w211:cluster{i32[], i32[]}[], "Numeric out"=w232:i32, "Boolean"=w212:bool)  [unwired: 1 in]
        n79 = case shown="True" "Apply Moving Average?" {
          tunnel: w202 -> [_ w264]
          frame False {
          }
          frame True {
            w262 = 3 ("side points")
            w263 = 1 ("polynomial order")
            n80 = Unbundle(w264) -> (w257:dbl, w253:dbl, w252:dbl)
            n81 = call <vilib>:"Savitzky Golay Filter PtByPt.vi"("order polynomial"=w263, "side points"=w262, "x"=w257) -> ("Filtered x"=w256:dbl)  [unwired: 1 in, 1 out]
            n82 = call <vilib>:"Savitzky Golay Filter PtByPt.vi"("order polynomial"=w263, "side points"=w262, "x"=w253) -> ("Filtered x"=w255:dbl)  [unwired: 1 in, 1 out]
            n83 = call <vilib>:"Savitzky Golay Filter PtByPt.vi"("order polynomial"=w263, "side points"=w262, "x"=w252) -> ("Filtered x"=w254:dbl)  [unwired: 1 in, 1 out]
            n84 = call <vilib>:"Derivative x(t) PtByPt.vi"("x"=w256) -> ("dx/dt"=w260:dbl)  [unwired: 3 in, 1 out]
            n85 = call <vilib>:"Derivative x(t) PtByPt.vi"("x"=w255) -> ("dx/dt"=w259:dbl)  [unwired: 3 in, 1 out]
            n86 = call <vilib>:"Derivative x(t) PtByPt.vi"("x"=w254) -> ("dx/dt"=w258:dbl)  [unwired: 3 in, 1 out]
            n87 = Bundle(w257, "Filtered x"=w256, w253, "Filtered x"=w255, w252, "Filtered x"=w254) -> (→"Thermocouple T-Plots":T4)  [unwired: 1 in]
            n88 = Bundle("dx/dt"=w260, "dx/dt"=w259, "dx/dt"=w258) -> (→"dT/dt":cluster{"dx/dt":dbl, "dx/dt":dbl, "dx/dt":dbl})  [unwired: 1 in]
          }
        }
        n89 = event shown="[1] \"STOP\": Value Change" {
          selector: _ -> [_ _]
          dyn-events: _ -> [_ _]
          timeout: 1000 -> [_ _]
          tunnel: [FALSE TRUE] -> w200
          event Timeout {
            n90 = event-data() -> ()  [unwired: 1 in, 3 out]
          }
          event "STOP": Value Change {
            n91 = event-data() -> ()  [unwired: 1 in, 5 out]
          }
        }
        n92 = case shown="True" w212 {
          tunnel: w211 -> [_ w285]
          frame False {
          }
          frame True {
            "Raman Spectrum" <- w285
          }
        }
        n93 = case shown="True" "Apply dF/dt?" {
          tunnel: w196 -> [_ w248]
          frame False {
          }
          frame True {
            n94 = Unbundle(w248) -> (w243:dbl, w244:dbl, w245:dbl, w246:dbl, w247:dbl)
            n95 = call <vilib>:"Derivative x(t) PtByPt.vi"("x"=w243) -> ("dx/dt"=w238:dbl)  [unwired: 3 in, 1 out]
            n96 = call <vilib>:"Derivative x(t) PtByPt.vi"("x"=w244) -> ("dx/dt"=w239:dbl)  [unwired: 3 in, 1 out]
            n97 = call <vilib>:"Derivative x(t) PtByPt.vi"("x"=w245) -> ("dx/dt"=w240:dbl)  [unwired: 3 in, 1 out]
            n98 = call <vilib>:"Derivative x(t) PtByPt.vi"("x"=w246) -> ("dx/dt"=w241:dbl)  [unwired: 3 in, 1 out]
            n99 = call <vilib>:"Derivative x(t) PtByPt.vi"("x"=w247) -> ("dx/dt"=w242:dbl)  [unwired: 3 in, 1 out]
            n100 = Bundle("dx/dt"=w238, "dx/dt"=w239, "dx/dt"=w240, "dx/dt"=w241, "dx/dt"=w242) -> (→"dF/dt":T20)  [unwired: 1 in]
          }
        }
        n101 = call "Julabo_Display_Values_subVI.vi"("VISA Refnum in"=w203) -> ("Safety Temp"=→"Safety Temp":dbl, "Excess Temp Protection"=→"Excess Temp Protection":dbl, "Power"=→"Power":i8, "Internal Temp"=→"Internal Temp":dbl, "External Temp"=→"External Temp":dbl, "Diagram"=→"Diagram":T8)  [unwired: 3 in, 2 out]
        n102 = case shown="True" "Write to File?" {
          tunnel: w219 -> [_ w284]
          tunnel: w215 -> [_ w283]
          tunnel: w196 -> [_ w282]
          tunnel: w230 -> [_ w277]
          tunnel: w229 -> [_ w276]
          tunnel: [w265 w271] -> w235
          tunnel: w223 -> [w265 w278]
          tunnel: [_ w277] -> w231
          tunnel: w211 -> [_ w275]
          tunnel: w224 -> [_ w274]
          tunnel: w218 -> [_ w273]
          tunnel: w204 -> [_ w272]
          frame False {
            # "eventually find more elegant way\nto do this - currently just an output on/off\nswitch for all intents and purposes"
          }
          frame True {
            n103 = Subtract(x=w277, y=w276) -> (x-y=w281:i32)
            n104 = Equal?(x=w281, y=1) -> (x = y?=w279:bool)
            n105 = call "File_Write_v2.vi"("Thermocouple Data"=w284, "Pressure Data"=w283, "Flow Rate Data"=w282, "Raman Data Array"=w275, "Loop Iteration Boolean"=w279, "Slave Data Cluster"=w272, "File Path Cluster"=w278, "Numeric"=w273, "Array"=w274) -> ("Filepath Cluster Out"=w271:T14)  [unwired: 13 in, 5 out]
            n106 = Unbundle By Name(w271) -> ("appended path"=→"Data_noRaman path":path, "appended path"=→"Data_Reactant 1 path":path, "appended path"=→"Data_Reactant 2 path":path, "appended path"=→"Data_Reactant 3 path":path, "appended path"=→"Data_Product path":path)
          }
        }
        "Measurement Iteration" <- w230
      }
      n107 = while {
        tunnel: w34 -> [w67]
        tunnel: w33 -> [w66]
        tunnel: w32 -> [w65]
        tunnel: w31 -> [w64]
        i -> [w61]
        stop <- w62 stop-if-true
        # "Producer"
        n108 = event shown="[2] \"STOP\": Value Change" {
          selector: _ -> [_ _ _ _ _ _ _ _ _ _ _ _ _ _ _ _ _ _ _ _ _]
          dyn-events: _ -> [_ _ _ _ _ _ _ _ _ _ _ _ _ _ _ _ _ _ _ _ _]
          timeout: u32 1000 ("Time") -> [_ _ _ _ _ _ _ _ _ _ _ _ _ _ _ _ _ _ _ _ _]
          tunnel: w65 -> [w70 w78 w83 w89 w92 w97 w103 w106 w110 w115 w118 w122 w128 w138 w144 w152 w160 w168 w176 w184 w192]
          tunnel: w64 -> [w71 w80 w85 w87 w93 w95 w102 w107 w109 w114 w119 w123 w130 w137 w145 w153 w161 w169 w177 w185 w193]
          tunnel: [w69 w79 w84 w86 w90 w94 w98 w105 w108 w112 _ w121 w129 w136 w146 w154 w162 w170 w178 w186 w194] -> _
          tunnel: [_ _ _ _ _ _ _ _ _ _ w117 _ _ _ _ _ _ _ _ _ _] -> _
          tunnel: [_ _ "STOP" _ _ _ _ _ _ _ _ _ _ _ _ _ _ _ _ _ _] -> w62
          tunnel: w66 -> [_ _ _ _ _ _ _ _ _ _ _ _ w126 w133 w141 w149 w157 w165 w174 w181 w189]
          tunnel: w67 -> [_ _ _ _ _ _ _ _ _ _ _ _ w124 w134 w140 w148 w156 w164 w175 w180 w188]
          tunnel: [_ _ _ _ _ _ _ _ _ _ _ _ w125 w132 w142 w150 w158 w166 w173 w182 w190] -> _
          event Timeout {
            n109 = event-data() -> ()  [unwired: 1 in, 2 out]
            n110 = case shown="False" FALSE {
              tunnel: w71 -> [w72 w76]
              tunnel: w70 -> [_ w75]
              tunnel: [w72 w73] -> w69
              frame False {
              }
              frame True {
                n111 = Enqueue Element(queue=w75, element="Idle", error in (no error)=w76) -> (error out=w73:errorcluster)  [unwired: 1 in, 2 out]
              }
            }
          }
          event "Set COMs": Value Change {
            n112 = event-data() -> ()  [unwired: 1 in, 6 out]
            n113 = Enqueue Element(queue=w78, element="SetCOMs", error in (no error)=w80) -> (error out=w79:errorcluster)  [unwired: 1 in, 2 out]
          }
          event "STOP": Value Change {
            n114 = event-data() -> ()  [unwired: 1 in, 6 out]
            n115 = Enqueue Element(queue=w83, element="stop", error in (no error)=w85) -> (error out=w84:errorcluster)  [unwired: 1 in, 2 out]
          }
          event "Run Current DoE": Value Change {
            n116 = event-data() -> ()  [unwired: 1 in, 5 out]
            n117 = Enqueue Element(queue=w89, element="Run DoE", error in (no error)=w87) -> (error out=w86:errorcluster)  [unwired: 1 in, 2 out]
          }
          event "Manual Pump Control?": Value Change {
            n118 = event-data() -> ()  [unwired: 1 in, 5 out]
            n119 = Enqueue Element(queue=w92, element="Manual Pump", error in (no error)=w93) -> (error out=w90:errorcluster)  [unwired: 1 in, 2 out]
          }
          event "Create DoE": Value Change {
            n120 = event-data() -> ()  [unwired: 1 in, 5 out]
            n121 = Enqueue Element(queue=w97, element="Create DoE", error in (no error)=w95) -> (error out=w94:errorcluster)  [unwired: 1 in, 2 out]
          }
          event "Cancel Script": Value Change {
            n122 = event-data() -> ()  [unwired: 1 in, 5 out]
            n123 = Flush Queue(queue=w103, error in (no error)=w102) -> (queue out=w101:refnum<queue>, error out=w100:errorcluster)  [unwired: 1 out]
            n124 = Enqueue Element(queue=w101, element="Abort", error in (no error)=w100) -> (error out=w98:errorcluster)  [unwired: 1 in, 2 out]
          }
          event "Manual Temp Control?": Value Change {
            n125 = event-data() -> ()  [unwired: 1 in, 5 out]
            n126 = Enqueue Element(queue=w106, element="Manual Temp", error in (no error)=w107) -> (error out=w105:errorcluster)  [unwired: 1 in, 2 out]
          }
          event "Load DoE": Value Change {
            n127 = event-data() -> ()  [unwired: 1 in, 5 out]
            n128 = Enqueue Element(queue=w110, element="Load DoE", error in (no error)=w109) -> (error out=w108:errorcluster)  [unwired: 1 in, 2 out]
          }
          event "Get Current DoE": Value Change {
            n129 = event-data() -> ()  [unwired: 1 in, 5 out]
            n130 = Enqueue Element(queue=w115, element="Get DoE", error in (no error)=w114) -> (error out=w112:errorcluster)  [unwired: 1 in, 2 out]
          }
          event "Debug": Value Change {
            n131 = event-data() -> ()  [unwired: 1 in, 5 out]
            n132 = Enqueue Element(queue=w118, element="Debugging / Send Command", error in (no error)=w119) -> (error out=w117:errorcluster)  [unwired: 1 in, 2 out]
          }
          event "Reset?": Value Change {
            n133 = event-data() -> ()  [unwired: 1 in, 5 out]
            n134 = Enqueue Element(queue=w122, element="Reset", error in (no error)=w123) -> (error out=w121:errorcluster)  [unwired: 1 in, 2 out]
          }
          event "btnAdjustWarningLevels": Value Change {
            n135 = event-data() -> ()  [unwired: 1 in, 6 out]
            n136 = Enqueue Element(queue=w124, element="JulaboAdjustWarningLevels", error in (no error)=w126) -> (error out=w125:errorcluster)  [unwired: 1 in, 2 out]
            n137 = Enqueue Element(queue=w128, element="JulaboControl", error in (no error)=w130) -> (error out=w129:errorcluster)  [unwired: 1 in, 2 out]
          }
          event "btnAdjustCapacityLevels": Value Change {
            n138 = event-data() -> ()  [unwired: 1 in, 6 out]
            n139 = Enqueue Element(queue=w134, element="JulaboAdjustCapacityLevels", error in (no error)=w133) -> (error out=w132:errorcluster)  [unwired: 1 in, 2 out]
            n140 = Enqueue Element(queue=w138, element="JulaboControl", error in (no error)=w137) -> (error out=w136:errorcluster)  [unwired: 1 in, 2 out]
          }
          event "btnAdjustInternalTempLimits": Value Change {
            n141 = event-data() -> ()  [unwired: 1 in, 6 out]
            n142 = Enqueue Element(queue=w144, element="JulaboControl", error in (no error)=w145) -> (error out=w146:errorcluster)  [unwired: 1 in, 2 out]
            n143 = Enqueue Element(queue=w140, element="JulaboAdjustInternalTempLimits", error in (no error)=w141) -> (error out=w142:errorcluster)  [unwired: 1 in, 2 out]
          }
          event "btnAdjustBandLimits": Value Change {
            n144 = event-data() -> ()  [unwired: 1 in, 6 out]
            n145 = Enqueue Element(queue=w152, element="JulaboControl", error in (no error)=w153) -> (error out=w154:errorcluster)  [unwired: 1 in, 2 out]
            n146 = Enqueue Element(queue=w148, element="JulaboAdjustBandLimits", error in (no error)=w149) -> (error out=w150:errorcluster)  [unwired: 1 in, 2 out]
          }
          event "btnAdjustInternalControlParams": Value Change {
            n147 = event-data() -> ()  [unwired: 1 in, 6 out]
            n148 = Enqueue Element(queue=w160, element="JulaboControl", error in (no error)=w161) -> (error out=w162:errorcluster)  [unwired: 1 in, 2 out]
            n149 = Enqueue Element(queue=w156, element="JulaboAdjustInternalControlParams", error in (no error)=w157) -> (error out=w158:errorcluster)  [unwired: 1 in, 2 out]
          }
          event "btnAdjustExternalControlParams": Value Change {
            n150 = event-data() -> ()  [unwired: 1 in, 6 out]
            n151 = Enqueue Element(queue=w168, element="JulaboControl", error in (no error)=w169) -> (error out=w170:errorcluster)  [unwired: 1 in, 2 out]
            n152 = Enqueue Element(queue=w164, element="JulaboAdjustExternalControlParams", error in (no error)=w165) -> (error out=w166:errorcluster)  [unwired: 1 in, 2 out]
          }
          event "JulaboStartStop": Value Change {
            n153 = event-data() -> ()  [unwired: 1 in, 6 out]
            n154 = Enqueue Element(queue=w176, element="JulaboControl", error in (no error)=w177) -> (error out=w178:errorcluster)  [unwired: 1 in, 2 out]
            n155 = Enqueue Element(queue=w175, element="JulaboStartStop", error in (no error)=w174) -> (error out=w173:errorcluster)  [unwired: 1 in, 2 out]
          }
          event "Julabo Control Type": Value Change {
            n156 = event-data() -> ()  [unwired: 1 in, 6 out]
            n157 = Enqueue Element(queue=w184, element="JulaboControl", error in (no error)=w185) -> (error out=w186:errorcluster)  [unwired: 1 in, 2 out]
            n158 = Enqueue Element(queue=w180, element="JulaboControlType", error in (no error)=w181) -> (error out=w182:errorcluster)  [unwired: 1 in, 2 out]
          }
          event "Julabo Setpoint": Value Change {
            n159 = event-data() -> ()  [unwired: 1 in, 6 out]
            n160 = Enqueue Element(queue=w192, element="JulaboControl", error in (no error)=w193) -> (error out=w194:errorcluster)  [unwired: 1 in, 2 out]
            n161 = Enqueue Element(queue=w188, element="JulaboSetPoint", error in (no error)=w189) -> (error out=w190:errorcluster)  [unwired: 1 in, 2 out]
          }
        }
        "Producer Iteration" <- w61
      }
      n162 = property on="Thermocouple T-Plots" class="WFChart (strict)"("History Data"=T15 []) -> ()  [unwired: 2 in, 2 out]
      n163 = property on="Flow Rate" class="WFChart (strict)"("History Data"=T16 []) -> ()  [unwired: 2 in, 2 out]
      n164 = property on="Temp" class="WFChart (strict)"("History Data"=T18 []) -> ()  [unwired: 2 in, 2 out]
      n165 = property on="Pressure" class="WFChart (strict)"("History Data"=T17 []) -> ()  [unwired: 2 in, 2 out]
      n166 = property on="Raman Spectrum" class="XYGraph (strict)"("Value"=cluster{i32[], i32[]}[] [] ("Raman Spectrum")) -> ()  [unwired: 2 in, 2 out]
      n167 = Release Queue(queue=w60) -> ()  [unwired: 2 in, 3 out]
      n168 = Release Queue(queue=w54) -> ()  [unwired: 2 in, 3 out]
    }
  }
